vi "Main.vi"(10 "DMM Port":refnum<visa-resource-name>, 11 "Module Admin":refnum<class "Delacor_lib_QMH_Module Admin.lvclass">) -> ()   [LabVIEW 2018, in "DMM Module.lvlib"]
doc: "This template is based off of the Queued Message Handler design pattern and the Queued Message Handler project template that ships with LabVIEW.\n\nThe main difference is that the queue is private to this module and communication between modules is performed via Broadcast and Request events.\n\nRequest events are wrapped in public API methods and are handled in the Event Handling Loop (EHL) of this VI. Any module can register for Broadcast events sent by this module. The EHL generates messages based on user interface actions.\n\nThe Message Handling Loop (MHL) processes messages generated by the EHL, or by other messages. The messages are string values, so new messages can be added easily to the Message Cases case structure in the MHL. Each message cluster can also provide an optional value for Message Data, which is a variant that can be converted to whatever message-specific data is required.\n_____\nBased on DQMH Project Template 6.0.0.91."
uses:
  DMM Module.lvlib
  <vilib>/Delacor/Delacor QMH/Libraries/Module Admin_class/Delacor_lib_QMH_Module Admin.lvclass
  Module Data--cluster.ctl
  config channel Argument--cluster.ctl
  <vilib>/Delacor/Delacor QMH/Libraries/Message Queue_class/Delacor_lib_QMH_Message Queue.lvclass/Delacor_lib_QMH_Message Queue.ctl
  DMM init Argument--cluster.ctl
  Read DCV_DCI Argument--cluster.ctl
  Read DCV_DCI (Reply Payload)--cluster.ctl
  DMM Close Argument--cluster.ctl
  DMM connect and reset Argument--cluster.ctl
  DMM reset Argument--cluster.ctl
  Stop Argument--cluster.ctl
  <vilib>/Delacor/Delacor QMH/Libraries/Module Admin_class/Delacor_lib_QMH_Module Admin.lvclass/Delacor_lib_QMH_Module Admin.ctl
  Query func Argument--cluster.ctl
  Query func (Reply Payload)--cluster.ctl
  query range Argument--cluster.ctl
  query range (Reply Payload)--cluster.ctl
  <vilib>/Utility/miscctls.llb/LVPointTypeDef.ctl
  <vilib>/Delacor/Delacor QMH/Libraries/Message Queue_class/Delacor_lib_QMH_Enqueue Message (Single).vi
  <vilib>/Delacor/Delacor QMH/Libraries/Module Admin_class/Delacor_lib_QMH_Get External Launch.vi
  <vilib>/Utility/error.llb/Error Cluster From Error Code.vi
  <vilib>/ErrorRing/Error Ring.xnode
  <vilib>/Delacor/Delacor QMH/Libraries/Message Queue_class/Delacor_lib_QMH_Message Queue.lvclass
  <instrlib>/DMM4/DMM4.lvlib
panel:
  in  "DMM reset":bool
  in  "Sets to Display":u16(ring)=2 items=["1st Display", "2nd Display", "1st & 2nd Display"]
  out "DCI":dbl
  out "DCV":dbl
  in  "Read DCV, DCI Dual mode":bool
  in  "Config Channel":bool
  in  "Detector Rate":u8(ring)=1 items=["SLOW", "MID", "FAST"]
  in  "DCI Range":dbl=1.0
  in  "DCV Range":dbl=1000.0
  in  "Open&Init":bool caption="Open&init"
  out "error out":errorcluster
  out "Status":string
  in  "Simulate MHL Error":bool
  in  "Simulate EHL Error":bool
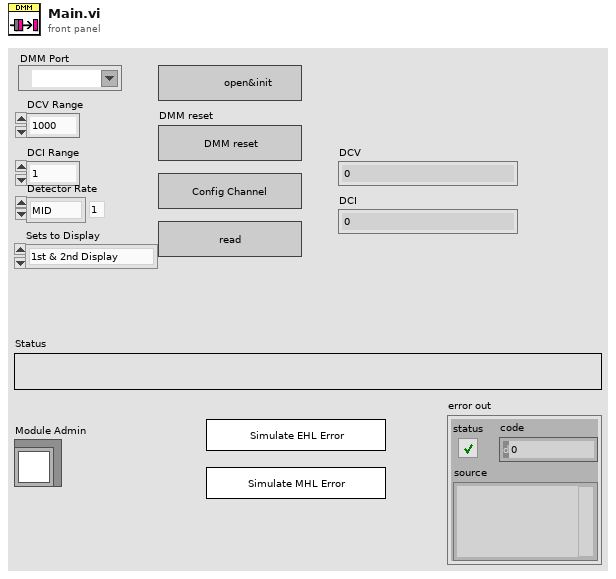
[diagram p1: front panel]
types:
  T1 = typedef "DMM Module.lvlib/Request Events--cluster.ctl" = cluster{"Stop Module":refnum<user-event>, "Do Something Else":refnum<user-event>, "Do Something Else and Wait for Reply":refnum<user-event>, "Show Panel":refnum<user-event>, "Hide Panel":refnum<user-event>, "Get Module Execution Status":refnum<user-event>, "Show Diagram":refnum<user-event>, "DMM init":refnum<user-event>, "config channel":refnum<user-event>, "Read DCV_DCI":refnum<user-event>, "DMM Close":refnum<user-event>, "DMM connect and reset":refnum<user-event>, "DMM reset":refnum<user-event>, "Query func":refnum<user-event>, "query range":refnum<user-event>}
  T2 = typedef "DMM Module.lvlib/Module Data--cluster.ctl" = cluster{"Status":string, "DMM  name":refnum<visa-resource-name>}
  T3 = typedef "DMM Module.lvlib/config channel Argument--cluster.ctl" = cluster{"Boolean":bool, "DCV range":dbl, "DCI range ":dbl, "Detector Rate":u8}
  T4 = typedef "DMM Module.lvlib/DMM init Argument--cluster.ctl" = cluster{"VISA resource name":refnum<visa-resource-name>}
  T5 = typedef "DMM Module.lvlib/Read DCV_DCI Argument--cluster.ctl" = cluster{"Wait Notifier":refnum<notifier>, "wait for reply":bool, "Sets to Display":u16}
  T6 = typedef "DMM Module.lvlib/DMM Close Argument--cluster.ctl" = cluster{"Boolean":bool}
  T7 = typedef "DMM Module.lvlib/DMM connect and reset Argument--cluster.ctl" = cluster{"Boolean":bool}
  T8 = typedef "DMM Module.lvlib/DMM reset Argument--cluster.ctl" = cluster{"Boolean":bool}
  T9 = enum32{"invalid lock state", "Not Locked", "Locked (No Password)", "Password-protected"}
  T10 = typedef "DMM Module.lvlib/Stop Argument--cluster.ctl" = cluster{"Origin":string, "Exit via Stop Module Req?":bool, "Wait for Module to stop?":bool}
  T11 = typedef "DMM Module.lvlib/Query func Argument--cluster.ctl" = cluster{"Wait Notifier":refnum<notifier>, "wait for reply":bool}
  T12 = typedef "DMM Module.lvlib/query range Argument--cluster.ctl" = cluster{"Wait Notifier":refnum<notifier>, "wait for reply":bool}
  T13 = typedef "LVPointTypeDef.ctl" = cluster{"Horizontal":i16, "Vertical":i16}
  T14 = enum32{"Invalid", "Standard", "Closed", "Hidden", "Minimized", "Maximized"}
  T15 = typedef "DMM Module.lvlib/Read DCV_DCI (Reply Payload)--cluster.ctl" = cluster{"DCV(Volts)":dbl, "DCI(mA)":dbl, "Read DCV_DCI_error":errorcluster}
  T16 = typedef "DMM Module.lvlib/Query func (Reply Payload)--cluster.ctl" = cluster{"String":string, "Query func_error":errorcluster}
  T17 = typedef "DMM Module.lvlib/query range (Reply Payload)--cluster.ctl" = cluster{"String":string, "query range_error":errorcluster}
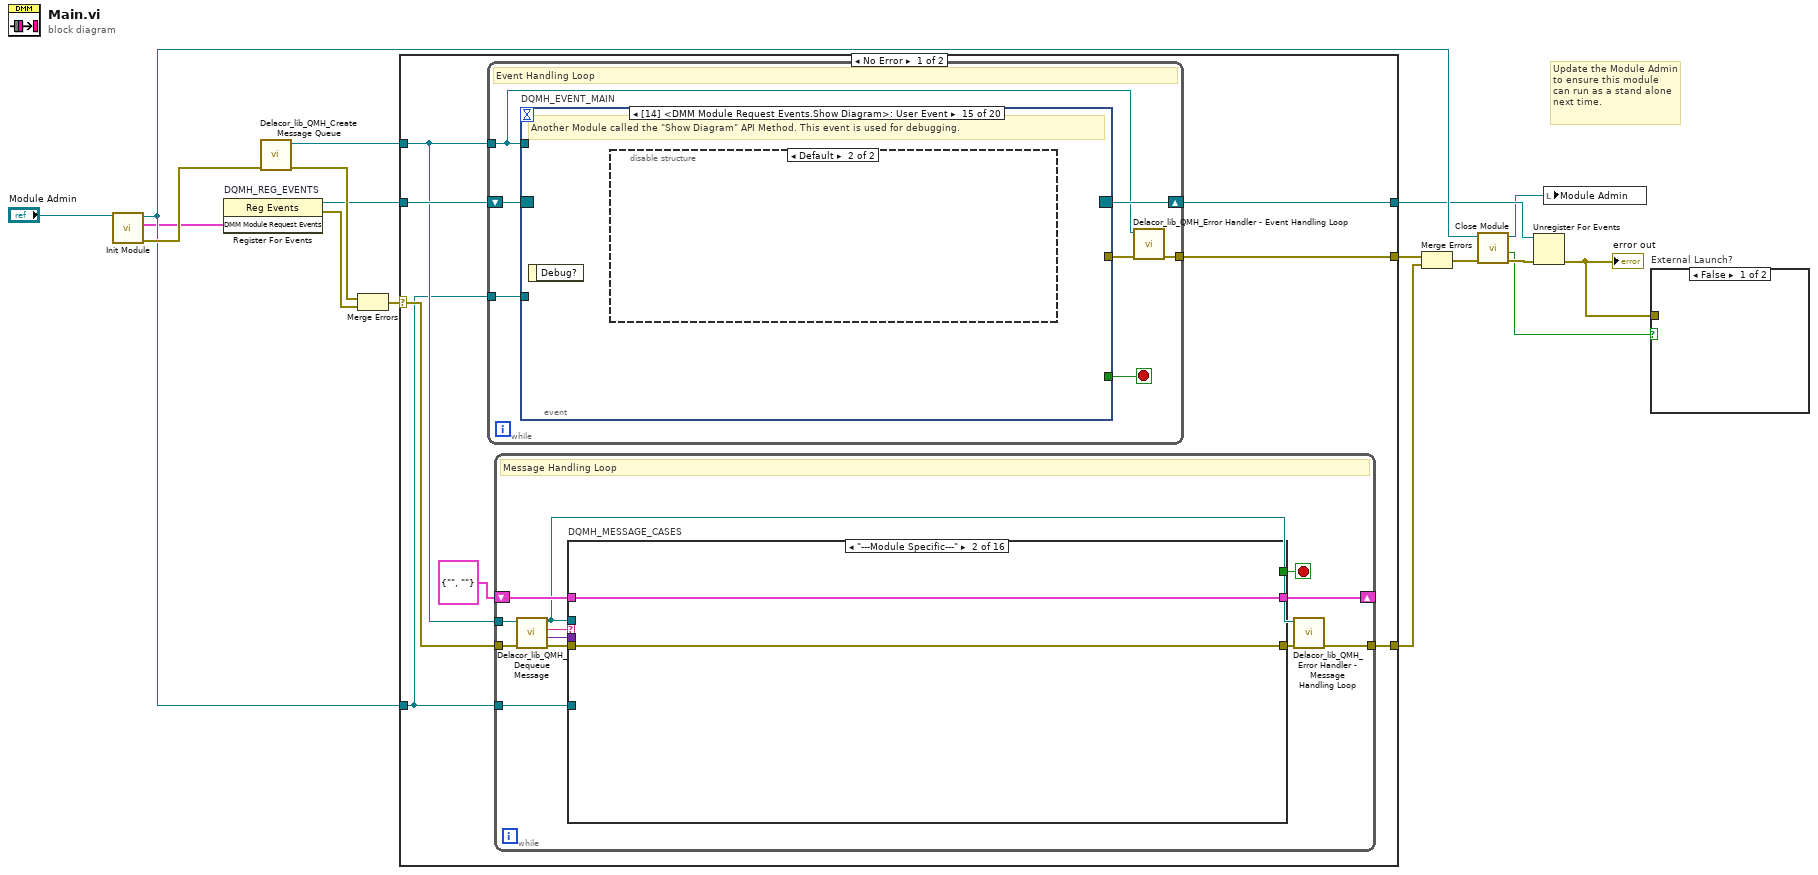
[diagram p0: block diagram]
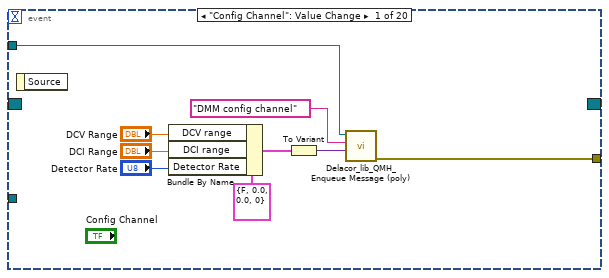
[diagram p2: hidden frame]
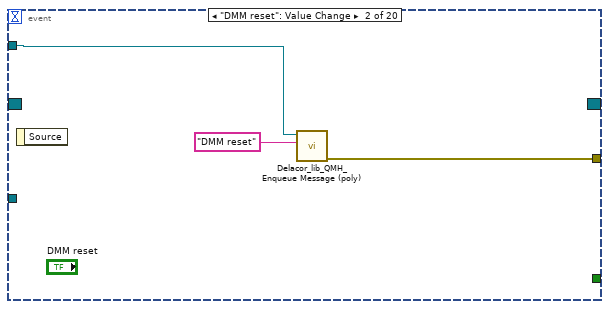
[diagram p3: hidden frame]
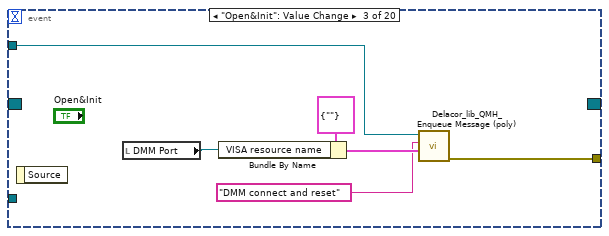
[diagram p4: hidden frame]
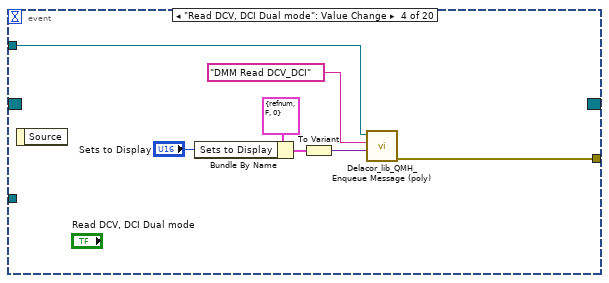
[diagram p5: hidden frame]
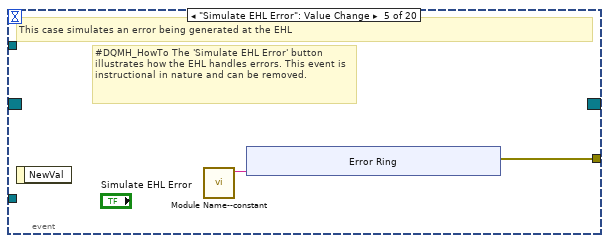
[diagram p6: hidden frame]
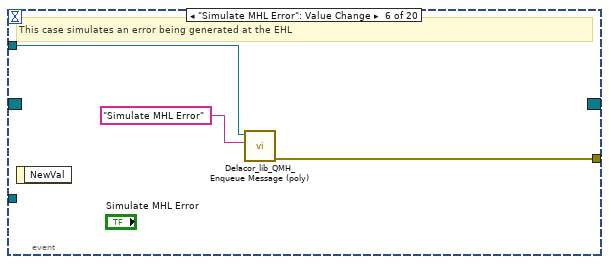
[diagram p7: hidden frame]
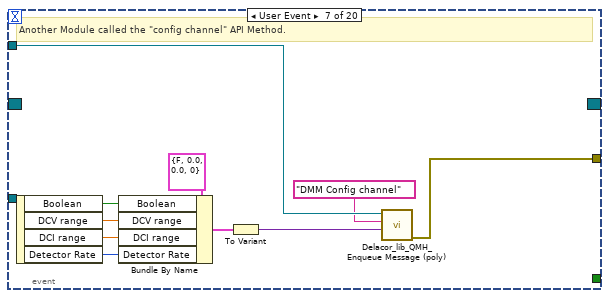
[diagram p8: hidden frame]
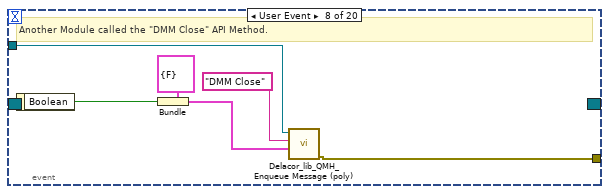
[diagram p9: hidden frame]
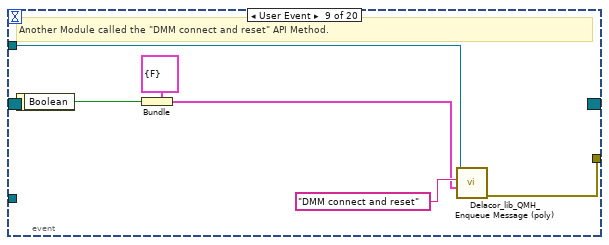
[diagram p10: hidden frame]
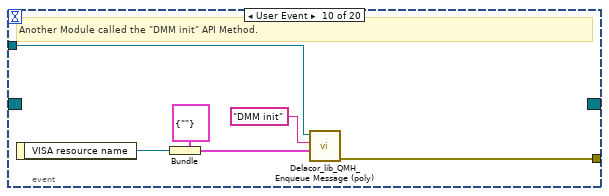
[diagram p11: hidden frame]
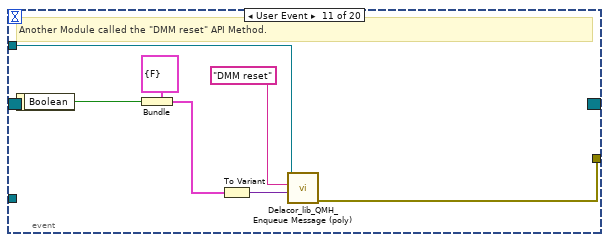
[diagram p12: hidden frame]
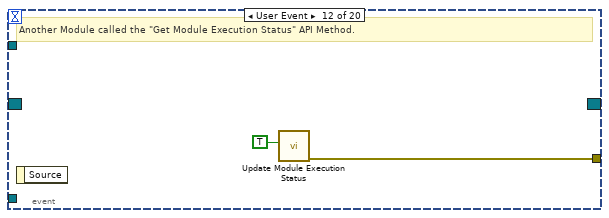
[diagram p13: hidden frame]
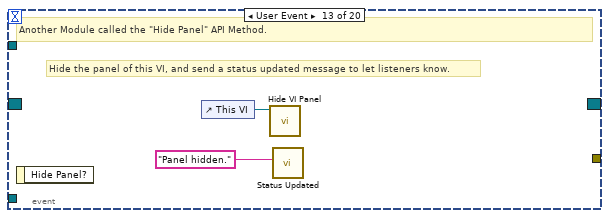
[diagram p14: hidden frame]
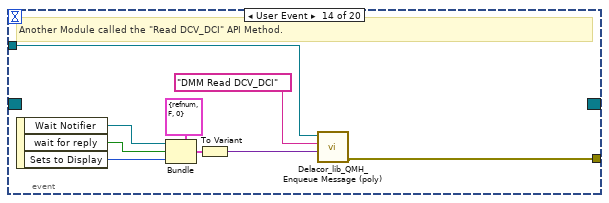
[diagram p15: hidden frame]
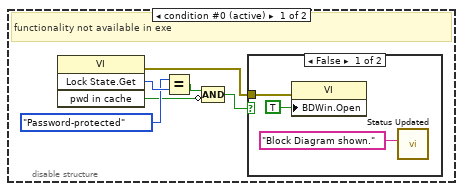
[diagram p16: hidden frame]
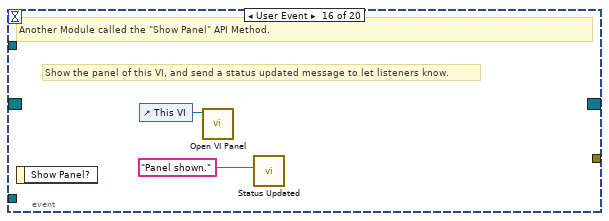
[diagram p18: hidden frame]
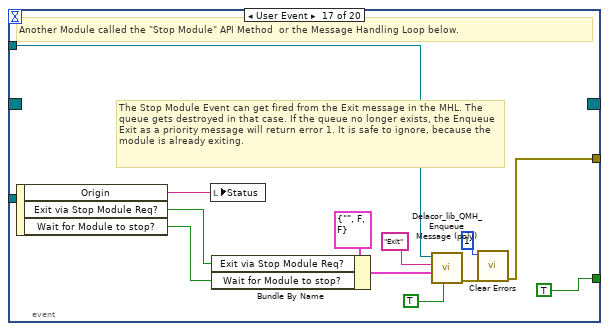
[diagram p19: hidden frame]
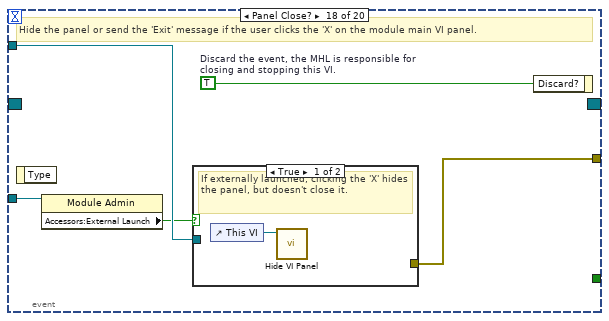
[diagram p20: hidden frame]
diagram:
  # "Update the Module Admin to ensure this module can run as a stand alone next time."
  n1 = call "Init Module.vi"("Singleton Module Admin in"="Module Admin") -> ("error out"=w16:errorcluster, "DMM Module Request Events"=w5:T1, "Singleton Module Admin out"=w8:refnum<class "Delacor_lib_QMH_Module Admin.lvclass">)  [unwired: 8 in]
  n2 = register-events "DQMH_REG_EVENTS"(w5) -> (reference out=w6:refnum<event-registration>, error out=w9:errorcluster)  [unwired: 2 in]
  n3 = call <vilib>:"Delacor_lib_QMH_Create Message Queue.vi"("error in"=w16) -> ("error out"=w11:errorcluster, "Message Queue"=w4:refnum<class "Delacor_lib_QMH_Message Queue.lvclass">)  [unwired: 9 in]
  n4 = Merge Errors(w11, w9) -> (w10:errorcluster)
  n5 = case shown="No Error" w10 {
    selector: w10 -> [w23 w418]
    tunnel: [w25 w417] -> w17
    tunnel: [w22 w423] -> w7
    tunnel: w6 -> [w20 w423]
    tunnel: w4 -> [w19 w416]
    tunnel: [w24 _] -> w14
    tunnel: w8 -> [w18 w419]
    frame No Error {
      n6 = while {
        tunnel: w19 -> [w26]
        shift-right: [w29] -> w22
        shift-left: w20 -> [w30]
        tunnel: [w31] -> w24
        tunnel: w18 -> [w27]
        stop <- w28 stop-if-true
        # "Event Handling Loop"
        n7 = event "DQMH_EVENT_MAIN" shown="[14] <DMM Module Request Events.Show Diagram>: User Event" {
          selector: w30 -> [_ _ _ _ _ _ _ _ _ _ _ _ _ _ _ _ _ _ _ _]
          dyn-events: [_ _ _ _ _ _ _ _ _ _ _ _ _ _ _ _ _ _ _ _] -> w29
          timeout: _ -> [_ _ _ _ _ _ _ _ _ _ _ _ _ _ _ _ _ _ _ _]
          tunnel: [_ _ _ _ _ _ _ _ _ _ _ _ _ _ _ _ TRUE ("Discard?") _ _ _] -> w28
          tunnel: w26 -> [w36 w44 w50 w57 _ w68 w79 w85 w91 w97 w104 _ _ w117 _ _ w129 w143 w157 w164]
          tunnel: [w35 w42 w47 w52 w59 w69 w75 w80 w86 w92 w100 w106 _ w111 _ _ w139 w145 w151 w158] -> w32
          tunnel: w27 -> [_ _ _ _ _ _ _ _ _ _ _ _ _ _ _ _ _ w142 _ _]
          event "Config Channel": Value Change {
            n8 = event-data() -> ()  [unwired: 1 in, 1 out]
            n9 = Bundle By Name(cluster=T3 {"Boolean"=FALSE, "DCV range"=0.0, "DCI range "=0.0, "Detector Rate"=0} ("config channel Argument"), "DCV range"="DCV Range", "DCI range"="DCI Range", "Detector Rate"="Detector Rate") -> (w34:T3)
            n10 = To Variant(anything=w34) -> (Variant=w33:variant)
            n11 = call-poly <vilib>:"Delacor_lib_QMH_Enqueue Message (poly).vi"("Message Data"=w33, "Message"="DMM config channel", "Message Queue in"=w36) -> ("error out"=w35:errorcluster)  [unwired: 7 in, 1 out]
          }
          event "DMM reset": Value Change {
            n12 = event-data() -> ()  [unwired: 1 in, 1 out]
            n13 = call-poly <vilib>:"Delacor_lib_QMH_Enqueue Message (poly).vi"("Message"="DMM reset", "Message Queue in"=w44) -> ("error out"=w42:errorcluster)  [unwired: 8 in, 1 out]
          }
          event "Open&Init": Value Change {
            n14 = event-data() -> ()  [unwired: 1 in, 1 out]
            n15 = local read "DMM Port"() -> (w46:refnum<visa-resource-name>)
            n16 = Bundle By Name(cluster=T4 {"VISA resource name"=""} ("DMM init Argument"), "VISA resource name"=w46) -> (w48:T4)
            n17 = call-poly <vilib>:"Delacor_lib_QMH_Enqueue Message (poly).vi"("Message Data"=w48, "Message"="DMM connect and reset", "Message Queue in"=w50) -> ("error out"=w47:errorcluster)  [unwired: 7 in, 1 out]
          }
          event "Read DCV, DCI Dual mode": Value Change {
            n18 = event-data() -> ()  [unwired: 1 in, 1 out]
            n19 = Bundle By Name(cluster=T5 {"Wait Notifier"=refnum, "wait for reply"=FALSE, "Sets to Display"=0} ("Read DCV_DCI Argument"), "Sets to Display"="Sets to Display") -> (w53:T5)
            n20 = To Variant(anything=w53) -> (Variant=w51:variant)
            n21 = call-poly <vilib>:"Delacor_lib_QMH_Enqueue Message (poly).vi"("Message Data"=w51, "Message"="DMM Read DCV_DCI", "Message Queue in"=w57) -> ("error out"=w52:errorcluster)  [unwired: 7 in, 1 out]
          }
          event "Simulate EHL Error": Value Change {
            # "#DQMH_HowTo The 'Simulate EHL Error' button  illustrates how the EHL handles errors. This event is instructional in nature and can be removed."
            # "This case simulates an error being generated at the EHL"
            n22 = event-data() -> ()  [unwired: 1 in, 1 out]
            n23 = call "Module Name--constant.vi"() -> ("Module Name"=w58:string)  [unwired: 11 in]
            n24 = xnode "Error Ring"("parameter 0"=w58) -> ("error out"=w59:errorcluster)
          }
          event "Simulate MHL Error": Value Change {
            # "This case simulates an error being generated at the EHL"
            n25 = event-data() -> ()  [unwired: 1 in, 1 out]
            n26 = call-poly <vilib>:"Delacor_lib_QMH_Enqueue Message (poly).vi"("Message"="Simulate MHL Error", "Message Queue in"=w68) -> ("error out"=w69:errorcluster)  [unwired: 8 in, 1 out]
          }
          event User Event {
            # "Another Module called the \"config channel\" API Method."
            n27 = event-data() -> ("Boolean"=w76:bool, "DCV range"=w74:dbl, "DCI range"=w73:dbl, "Detector Rate"=w72:u8)  [unwired: 1 in]
            n28 = Bundle By Name(cluster=T3 {"Boolean"=FALSE, "DCV range"=0.0, "DCI range "=0.0, "Detector Rate"=0} ("config channel Argument"), "Boolean"=w76, "DCV range"=w74, "DCI range"=w73, "Detector Rate"=w72) -> (w71:T3)
            n29 = To Variant(anything=w71) -> (Variant=w70:variant)
            n30 = call-poly <vilib>:"Delacor_lib_QMH_Enqueue Message (poly).vi"("Message Data"=w70, "Message"="DMM Config channel", "Message Queue in"=w79) -> ("error out"=w75:errorcluster)  [unwired: 7 in, 1 out]
          }
          event User Event {
            # "Another Module called the \"DMM Close\" API Method."
            n31 = event-data() -> ("Boolean"=w81:bool)  [unwired: 1 in]
            n32 = Bundle(cluster=T6 {"Boolean"=FALSE} ("DMM Close Argument"), "Boolean"=w81) -> (w82:T6)
            n33 = call-poly <vilib>:"Delacor_lib_QMH_Enqueue Message (poly).vi"("Message Data"=w82, "Message"="DMM Close", "Message Queue in"=w85) -> ("error out"=w80:errorcluster)  [unwired: 7 in, 1 out]
          }
          event User Event {
            # "Another Module called the \"DMM connect and reset\" API Method."
            n34 = event-data() -> ("Boolean"=w87:bool)  [unwired: 1 in]
            n35 = Bundle(cluster=T7 {"Boolean"=FALSE} ("DMM connect and reset Argument"), "Boolean"=w87) -> (w88:T7)
            n36 = call-poly <vilib>:"Delacor_lib_QMH_Enqueue Message (poly).vi"("Message Data"=w88, "Message"="DMM connect and reset", "Message Queue in"=w91) -> ("error out"=w86:errorcluster)  [unwired: 7 in, 1 out]
          }
          event User Event {
            # "Another Module called the \"DMM init\" API Method."
            n37 = event-data() -> ("VISA resource name"=w93:refnum<visa-resource-name>)  [unwired: 1 in]
            n38 = Bundle(cluster=T4 {"VISA resource name"=""} ("DMM init Argument"), "VISA resource name"=w93) -> (w94:T4)
            n39 = call-poly <vilib>:"Delacor_lib_QMH_Enqueue Message (poly).vi"("Message Data"=w94, "Message"="DMM init", "Message Queue in"=w97) -> ("error out"=w92:errorcluster)  [unwired: 7 in, 1 out]
          }
          event User Event {
            # "Another Module called the \"DMM reset\" API Method."
            n40 = event-data() -> ("Boolean"=w101:bool)  [unwired: 1 in]
            n41 = Bundle(cluster=T8 {"Boolean"=FALSE} ("DMM reset Argument"), "Boolean"=w101) -> (w99:T8)
            n42 = To Variant(anything=w99) -> (Variant=w98:variant)
            n43 = call-poly <vilib>:"Delacor_lib_QMH_Enqueue Message (poly).vi"("Message Data"=w98, "Message"="DMM reset", "Message Queue in"=w104) -> ("error out"=w100:errorcluster)  [unwired: 7 in, 1 out]
          }
          event User Event {
            # "Another Module called the \"Get Module Execution Status\" API Method."
            n44 = event-data() -> ()  [unwired: 1 in, 1 out]
            n45 = call "Update Module Execution Status.vi"("Running?"=TRUE) -> ("error out"=w106:errorcluster)  [unwired: 10 in]
          }
          event User Event {
            # "Hide the panel of this VI, and send a status updated message to let listeners know."
            # "Another Module called the \"Hide Panel\" API Method."
            n46 = event-data() -> ()  [unwired: 1 in, 1 out]
            n47 = control-ref of="This VI"() -> (w108:refnum<vi>)
            n48 = call "Hide VI Panel.vi"("VI"=w108) -> ()  [unwired: 10 in, 1 out]
            n49 = call "Status Updated.vi"("Status"="Panel hidden." ("format string")) -> ()  [unwired: 10 in, 1 out]
          }
          event User Event {
            # "Another Module called the \"Read DCV_DCI\" API Method."
            n50 = event-data() -> ("Wait Notifier"=w113:refnum<notifier>, "wait for reply"=w112:bool, "Sets to Display"=w110:u16)  [unwired: 1 in]
            n51 = Bundle(cluster=T5 {"Wait Notifier"=refnum, "wait for reply"=FALSE, "Sets to Display"=0} ("Read DCV_DCI Argument"), "Wait Notifier"=w113, "wait for reply"=w112, "Sets to Display"=w110) -> (w114:T5)
            n52 = To Variant(anything=w114) -> (Variant=w109:variant)
            n53 = call-poly <vilib>:"Delacor_lib_QMH_Enqueue Message (poly).vi"("Message Data"=w109, "Message"="DMM Read DCV_DCI", "Message Queue in"=w117) -> ("error out"=w111:errorcluster)  [unwired: 7 in, 1 out]
          }
          event User Event {
            # "Another Module called the \"Show Diagram\" API Method. This event is used for debugging."
            n54 = event-data() -> ()  [unwired: 1 in, 1 out]
            n55 = disable-structure shown="Default" {
              frame condition #0 (active) {
                # "functionality not available in exe"
                n56 = invoke class="VI" method="Lock State.Get"() -> (error out=w123:errorcluster, "Get Lock State"=w122:T9, "pwd in cache"=w119:bool)  [unwired: 4 in, 1 out]
                n57 = Equal?(x=T9."Password-protected", y=w122) -> (x = y?=w120:bool)
                n58 = Compound Arithmetic op=AND(w120, invert w119) -> (w118:bool)
                n59 = case shown="False" w118 {
                  tunnel: w123 -> [w126 _]
                  frame False {
                    n60 = property class="VI"(error in=w126, "BDWin.Open"=TRUE ("Block Diagram Window:Open")) -> ()  [unwired: 1 in, 2 out]
                    n61 = call "Status Updated.vi"("Status"="Block Diagram shown." ("format string")) -> ()  [unwired: 10 in, 1 out]
                  }
                  frame True {
                    # "Password-protected VI, and the password is not in the cache. Do not show the diagram."
                  }
                }
              }
              frame condition #1 {
              }
            }
          }
          event User Event {
            # "Show the panel of this VI, and send a status updated message to let listeners know."
            # "Another Module called the \"Show Panel\" API Method."
            n62 = event-data() -> ()  [unwired: 1 in, 1 out]
            n63 = control-ref of="This VI"() -> (w128:refnum<vi>)
            n64 = call "Open VI Panel.vi"("VI"=w128) -> ()  [unwired: 10 in, 1 out]
            n65 = call "Status Updated.vi"("Status"="Panel shown." ("format string")) -> ()  [unwired: 10 in, 1 out]
          }
          event User Event {
            # "The Stop Module Event can get fired from the Exit message in the MHL. The queue gets destroyed in that case. If the queue no longer exists, the Enqueue Exit as a priority message will return error 1. It is safe to ignore, because the module is already exiting."
            # "Another Module called the \"Stop Module\" API Method  or the Message Handling Loop below."
            n66 = event-data() -> ("Origin"=w136:string, "Exit via Stop Module Req?"=w132:bool, "Wait for Module to stop?"=w131:bool)  [unwired: 1 in]
            n67 = local write "Status"(w136) -> ()
            n68 = Bundle By Name(cluster=T10 {"Origin"="", "Exit via Stop Module Req?"=FALSE, "Wait for Module to stop?"=FALSE} ("Stop Argument"), "Exit via Stop Module Req?"=w132, "Wait for Module to stop?"=w131) -> (w130:T10)
            n69 = call-poly <vilib>:"Delacor_lib_QMH_Enqueue Message (poly).vi"("Priority Message? (F)"=TRUE, "Message Data"=w130, "Message"="Exit", "Message Queue in"=w129) -> ("error out"=w140:errorcluster)  [unwired: 6 in, 1 out]
            n70 = call <vilib>:"Clear Errors.vi"("error in (no error)"=w140, "specific error code to clear (0: all)"=1) -> ("error out"=w139:errorcluster)  [unwired: 4 in, 1 out]
          }
          event Panel Close? {
            w144 = TRUE  # Discard the event, the MHL is responsible for closing and stopping this VI.
            # "Hide the panel or send the 'Exit' message if the user clicks the 'X' on the module main VI panel."
            n71 = event-data() -> ()  [unwired: 1 in, 1 out]
            n72 = property class="Module Admin"(reference=w142) -> ("Accessors:External Launch"=w141:bool)  [unwired: 1 in, 2 out]
            n73 = case shown="True" w141 {
              tunnel: w143 -> [_ w149]
              tunnel: [_ w150] -> w145
              frame True {
                # "If externally launched, clicking the 'X' hides the panel, but doesn't close it."
                n74 = control-ref of="This VI"() -> (w146:refnum<vi>)
                n75 = call "Hide VI Panel.vi"("VI"=w146) -> ()  [unwired: 10 in, 1 out]
              }
              frame False {
                # "If run as a stand-alone VI, clicking the panel 'X' stops the VI."
                n76 = call-poly <vilib>:"Delacor_lib_QMH_Enqueue Message (poly).vi"("Priority Message? (F)"=TRUE, "Message"="Exit", "Message Queue in"=w149) -> ("error out"=w150:errorcluster)  [unwired: 7 in, 1 out]
              }
            }
            n77 = event-data("Discard?"=w144) -> ()  [unwired: 1 in, 1 out]
          }
          event User Event {
            # "Another Module called the \"Query func\" API Method."
            n78 = event-data() -> ("Wait Notifier"=w153:refnum<notifier>, "wait for reply"=w152:bool)  [unwired: 1 in]
            n79 = Bundle(cluster=T11 {"Wait Notifier"=refnum, "wait for reply"=FALSE} ("Query func Argument"), "Wait Notifier"=w153, "wait for reply"=w152) -> (w154:T11)
            n80 = call-poly <vilib>:"Delacor_lib_QMH_Enqueue Message (poly).vi"("Message Data"=w154, "Message"="Query func", "Message Queue in"=w157) -> ("error out"=w151:errorcluster)  [unwired: 7 in, 1 out]
          }
          event User Event {
            # "Another Module called the \"query range\" API Method."
            n81 = event-data() -> ("Wait Notifier"=w160:refnum<notifier>, "wait for reply"=w159:bool)  [unwired: 1 in]
            n82 = Bundle(cluster=T12 {"Wait Notifier"=refnum, "wait for reply"=FALSE} ("query range Argument"), "Wait Notifier"=w160, "wait for reply"=w159) -> (w161:T12)
            n83 = call-poly <vilib>:"Delacor_lib_QMH_Enqueue Message (poly).vi"("Message Data"=w161, "Message"="query range", "Message Queue in"=w164) -> ("error out"=w158:errorcluster)  [unwired: 7 in, 1 out]
          }
        }
        n84 = call-dynamic "Delacor_lib_QMH_Error Handler - Event Handling Loop.vi"("error in"=w32, "Message Queue in"=w26) -> ("dup error in"=w31:errorcluster)  [unwired: 8 in, 1 out]
      }
      n85 = while {
        tunnel: w19 -> [w167]
        shift-right: [w171] -> _
        shift-left: T2 {"Status"="", "DMM  name"=""} ("Data Cluster") -> [w172]
        tunnel: w23 -> [w175]
        tunnel: [w173] -> w25
        tunnel: w18 -> [w165]
        stop <- w170 stop-if-true
        # "Message Handling Loop"
        n86 = call-dynamic "Delacor_lib_QMH_Dequeue Message.vi"("error in"=w175, "Message Queue in"=w167) -> ("error out"=w174:errorcluster, "Message Data"=w168:variant, "Message"=w169:string, "Message Queue out"=w166:refnum<class "Delacor_lib_QMH_Message Queue.lvclass">)  [unwired: 6 in]
        n87 = case "DQMH_MESSAGE_CASES" shown="\"---Module Specific---\"" w169 {
          selector: w169 -> [_ _ _ _ _ _ _ _ _ _ _ _ _ _ _ w403]
          tunnel: w166 -> [_ _ _ _ _ _ _ _ _ _ _ _ _ w368 w390 _]
          tunnel: w174 -> [w195 w199 w206 w222 w232 w241 w257 w288 w325 w346 w349 w352 w357 w374 w396 w405]
          tunnel: [w179 w199 w201 w217 w229 w234 w253 w279 w316 w337 w349 w352 w356 w371 w393 w406] -> w176
          tunnel: w172 -> [w181 w198 w203 w219 w228 w237 w247 w278 w315 w336 w350 w351 w354 w370 w382 w404]
          tunnel: [w177 w198 w203 w219 w228 w237 w247 w278 w315 w336 w350 w351 w354 w370 w382 w404] -> w171
          tunnel: [_ _ _ _ _ _ _ _ _ _ _ _ _ _ w389 _] -> w170
          tunnel: w168 -> [_ _ w205 w221 w231 w240 w256 w286 w323 w344 _ _ _ w369 w388 _]
          tunnel: w165 -> [w188 _ _ _ _ _ _ _ _ _ _ _ _ w367 w383 _]
          frame "Initialize" {
            w178 = "Initial Message" ("Initial Message")
            # "Initialize - Any operation that needs to be done before the module can receive messages. Synchronize Caller Events.vi will inform Start Module.vi that the module has launched and is ready to receive messages. Module Did Init.vi will broadcast that the module initialized."
            n88 = call "Synchronize Caller Events.vi"("error in (no error)"=w195, "Singleton Module Admin in"=w188) -> ("error out"=w183:errorcluster, "Singleton Module Admin out"=w185:refnum<class "Delacor_lib_QMH_Module Admin.lvclass">)  [unwired: 8 in]
            n89 = property class="Module Admin"(reference=w185) -> ("Accessors:External Launch"=w182:bool)  [unwired: 1 in, 2 out]
            n90 = call "Module Name--constant.vi"() -> ("Module Name"=w194:string)  [unwired: 11 in]
            n91 = Select(t=T14."Hidden" ("State"), s=w182, f=T14."Standard" ("State")) -> (s? t:f=w189:T14)
            n92 = property class="VI"("Front Panel.Title"=w194) -> (reference out=w193:refnum<vi>, error out=w197:errorcluster)  [unwired: 2 in]
            n93 = invoke class="VI" method="FP.Open"(reference=w193, error in=w197, "State"=w189) -> (reference out=w192:refnum<vi>, error out=w196:errorcluster)  [unwired: 2 in, 3 out]
            n94 = Bundle By Name(cluster=w181, "DMM  name"="DMM Port", "Status"=w178) -> (w177:T2)
            n95 = invoke class="VI" method="FP.Center"(reference=w192, error in=w196) -> ()  [unwired: 1 in, 3 out]
            n96 = property on="Pane" class="Pane"("Origin"=T13 {"Horizontal"=0, "Vertical"=0}) -> ()  [unwired: 2 in, 2 out]
            n97 = call "Module Name--constant.vi"() -> ("Module Name"=w186:string)  [unwired: 11 in]
            n98 = call "Module Did Init.vi"("error in (no error)"=w183, "Initialized?"=TRUE, "Origin"=w186) -> ("error out"=w179:errorcluster)  [unwired: 8 in]
            "Status" <- w178
          }
          frame "---Module Specific---" {
            # "Separator -- The following cases handle messages specific to this Module."
          }
          frame "DMM connect and reset" {
            # "Connect DMM and reset DMM"
            n99 = Variant To Data(error in=w206, type=T7 {"Boolean"=FALSE} ("DMM connect and reset Argument"), Variant=w205) -> (error out=w202:errorcluster)  [unwired: 1 out]
            n100 = disable-structure shown="Default" {
              disable-tunnel: w203 -> [w210 _]
              disable-tunnel: [w208 _] -> w200
              frame condition #0 (active) {
                w211 = u32 115200 items=["9600"=9600, "19200"=19200, "38400"=38400, "57600"=57600, "115200"=115200] ("Configure RS232 Baud Rate")
                n101 = Unbundle By Name(w210) -> ("DMM  name"=w209:refnum<visa-resource-name>)
                n102 = call <instrlib>:"Initialize.vi"("Configure RS232 Baud Rate"=w211, "VISA resource name"=w209) -> ("error out"=w213:errorcluster, "VISA resource name out"=w212:refnum<visa-resource-name>)  [unwired: 6 in, 2 out]
                n103 = call <instrlib>:"Reset.vi"("error in (no error)"=w213, "VISA resource name"=w212) -> ("error out"=w207:errorcluster)  [unwired: 8 in, 1 out]
                n104 = flat-sequence {
                  tunnel: [w214] -> w208
                  tunnel: w207 -> [w214]
                  frame #0 {
                    n105 = Wait (ms)(milliseconds to wait=u32 200) -> ()  [unwired: 1 out]
                  }
                }
              }
              frame condition #1 {
              }
            }
            n106 = Merge Errors(w202, w200) -> (w201:errorcluster)
          }
          frame "DMM Close" {
            # "Close COMport to DMM"
            n107 = disable-structure shown="Default" {
              disable-tunnel: w219 -> [w227 _]
              disable-tunnel: [w226 _] -> w216
              frame condition #0 (active) {
                n108 = Unbundle By Name(w227) -> ("DMM  name"=w225:refnum<visa-resource-name>)
                n109 = call <instrlib>:"Reset.vi"("VISA resource name"=w225) -> ("error out"=w223:errorcluster, "VISA resource name out"=w224:refnum<visa-resource-name>)  [unwired: 9 in]
                n110 = call <instrlib>:"Close.vi"("error in (no error)"=w223, "VISA resource name"=w224) -> ("error out"=w226:errorcluster)  [unwired: 9 in]
              }
              frame condition #1 {
              }
            }
            n111 = Variant To Data(error in=w222, type=T6 {"Boolean"=FALSE} ("DMM Close Argument"), Variant=w221) -> (error out=w218:errorcluster)  [unwired: 1 out]
            n112 = Merge Errors(w218, w216) -> (w217:errorcluster)
          }
          frame "DMM init" {
            # "#Hung_comment :\nNo longer use"
            # "Open port and initialize DMM  and reset DMM"
            n113 = Variant To Data(error in=w232, type=T4 {"VISA resource name"=""} ("DMM init Argument"), Variant=w231) -> (error out=w229:errorcluster)  [unwired: 1 out]
          }
          frame "DMM reset" {
            # "Reset Measurement Mode"
            n114 = Variant To Data(error in=w241, type=T8 {"Boolean"=FALSE} ("DMM reset Argument"), Variant=w240) -> (data=w238:T8, error out=w236:errorcluster)
            n115 = Unbundle By Name(w238) -> ()  [unwired: 1 out]
            n116 = disable-structure shown="Default" {
              disable-tunnel: w237 -> [w244 _]
              disable-tunnel: [w242 _] -> w235
              frame condition #0 (active) {
                n117 = Unbundle By Name(w244) -> ("DMM  name"=w243:refnum<visa-resource-name>)
                n118 = call <instrlib>:"Reset.vi"("VISA resource name"=w243) -> ("error out"=w242:errorcluster)  [unwired: 9 in, 1 out]
              }
              frame condition #1 {
              }
            }
            n119 = Merge Errors(w236, w235) -> (w233:errorcluster)
            n120 = flat-sequence {
              tunnel: [w246] -> w234
              tunnel: w233 -> [w246]
              frame #0 {
                n121 = Wait (ms)(milliseconds to wait=u32 200) -> ()  [unwired: 1 out]
              }
            }
          }
          frame "DMM Config channel" {
            # "Config DMM mode: dual measurements, CH1: DCV; CH2: DCI"
            n122 = Variant To Data(error in=w257, type=T3 {"Boolean"=FALSE, "DCV range"=0.0, "DCI range "=0.0, "Detector Rate"=0} ("config channel Argument"), Variant=w256) -> (data=w254:T3, error out=w249:errorcluster)
            n123 = Unbundle By Name(w254) -> ("Detector Rate"=w250:u8, "DCV range"=w252:dbl, "DCI range"=w251:dbl)
            n124 = disable-structure shown="Default" {
              disable-tunnel: w252 -> [w272 _]
              disable-tunnel: w251 -> [w261 _]
              disable-tunnel: w250 -> [w270 _]
              disable-tunnel: [w258 _] -> w248
              disable-tunnel: w247 -> [w264 _]
              frame condition #0 (active) {
                w262 = FALSE ("Enable Auto Range")
                w260 = u8 2 items=["DC Voltage", "AC Voltage", "DC Current", "AC Current", "2-Wire Resistance", "Frequency", "Period", "None"] ("Function")
                w266 = u8 0 items=["DC Voltage", "AC Voltage", "DC+AC Voltage", "DC Current", "AC Current", "DC+AC Current", "2-Wire Resistance", "Frequency", "Period", "Continuity", "Diode", "Temperature", "Capacitance"] ("Function")
                n125 = Unbundle By Name(w264) -> ("DMM  name"=w271:refnum<visa-resource-name>)
                n126 = call <instrlib>:"Sets and Query the Detector Rate.vi"("Enable to Query"=FALSE, "Enable to Sets"=TRUE, "Detector Rate"=w270, "VISA resource name"=w271) -> ("error out"=w265:errorcluster, "VISA resource name out"=w267:refnum<visa-resource-name>)  [unwired: 5 in, 1 out]
                n127 = call <instrlib>:"Configure the Function on 1st Display .vi"("Manual Range"=w272, "Enable Auto Range"=w262, "error in"=w265, "Function"=w266, "VISA resource name"=w267) -> ("error out"=w259:errorcluster, "VISA resource name out"=w263:refnum<visa-resource-name>)  [unwired: 5 in]
                n128 = call <instrlib>:"Configure the Function on 2nd Display.vi"("Manual Range"=w261, "Enable Auto Range"=w262, "error in"=w259, "Function"=w260, "VISA resource name"=w263) -> ("error out"=w258:errorcluster)  [unwired: 5 in, 1 out]
              }
              frame condition #1 {
              }
            }
            n129 = Merge Errors(w249, w248) -> (w253:errorcluster)
          }
          frame "DMM Read DCV_DCI" {
            # "Read DCV, DCI dual measurements"
            n130 = Variant To Data(error in=w288, type=T5 {"Wait Notifier"=refnum, "wait for reply"=FALSE, "Sets to Display"=0} ("Read DCV_DCI Argument"), Variant=w286) -> (data=w284:T5, error out=w287:errorcluster)
            n131 = Unbundle By Name(w284) -> ("Sets to Display"=w276:u16, "Wait Notifier"=w283:refnum<notifier>, "wait for reply"=w282:bool)
            n132 = Unbundle By Name(w278) -> ("DMM  name"=w277:refnum<visa-resource-name>)
            n133 = disable-structure shown="Default" {
              disable-tunnel: w277 -> [w300 _]
              disable-tunnel: w276 -> [w299 _]
              disable-tunnel: [w298 _] -> w275
              disable-tunnel: [w294 128.09] -> w274
              disable-tunnel: [w289 292.0] -> w273
              frame condition #0 (active) {
                n134 = call <instrlib>:"Returns 1st and 2nd Display Value.vi"("Sets to Display"=w299, "VISA resource name"=w300) -> ("error out"=w298:errorcluster, "Return the Value"=w296:string)  [unwired: 7 in, 1 out]
                n135 = Match Pattern(string=w296, regular expression=",") -> (before substring=w295:string, after substring=w293:string)  [unwired: 1 in, 2 out]
                n136 = Fract/Exp String To Number(string=w295) -> (number=w294:dbl)  [unwired: 3 in, 1 out]
                "DCV" <- w294
                n137 = Fract/Exp String To Number(string=w293) -> (number=w292:dbl)  [unwired: 3 in, 1 out]
                "DCI" <- w292
                n138 = Multiply(x=w292, y=1000.0) -> (x*y=w290:dbl)
                n139 = Absolute Value(x=w290) -> (abs(x)=w289:dbl)
              }
              frame condition #1 {
              }
            }
            n140 = Merge Errors(w287, w275) -> (w279:errorcluster)
            n141 = Bundle By Name(cluster=T15 {"DCV(Volts)"=0.0, "DCI(mA)"=0.0, "Read DCV_DCI_error"={"status"=FALSE, "code"=0, "source"=""}} ("Read DCV_DCI (Reply Payload)"), "DCV(Volts)"=w274, "DCI(mA)"=w273) -> (w281:T15)
            n142 = case shown="True" w282 {
              tunnel: w283 -> [_ w304]
              tunnel: w281 -> [_ w303]
              frame False {
              }
              frame True {
                n143 = Send Notification(notification=w303, notifier=w304) -> ()  [unwired: 1 in, 2 out]
              }
            }
          }
          frame "Query func" {
            w306 = u8 1 items=["1st Display", "2nd Display"] ("Query form Display")
            w313 = u8 0 items=["1st Display", "2nd Display"] ("Query form Display")
            # "Check measurement Mode  chan1"
            n144 = Variant To Data(error in=w325, type=T11 {"Wait Notifier"=refnum, "wait for reply"=FALSE} ("Query func Argument"), Variant=w323) -> (data=w321:T11, error out=w324:errorcluster)
            n145 = Unbundle By Name(w315) -> ("DMM  name"=w314:refnum<visa-resource-name>)
            n146 = Unbundle By Name(w321) -> ("Wait Notifier"=w320:refnum<notifier>, "wait for reply"=w319:bool)
            n147 = call <instrlib>:"Query the Current Function.vi"("Query form Display"=w313, "VISA resource name"=w314) -> ("error out"=w312:errorcluster, "Return the String"=w310:string, "VISA resource name out"=w311:refnum<visa-resource-name>)  [unwired: 7 in]
            n148 = call <instrlib>:"Query the Current Function.vi"("error in"=w312, "Query form Display"=w306, "VISA resource name"=w311) -> ("error out"=w305:errorcluster, "Return the String"=w308:string)  [unwired: 6 in, 1 out]
            n149 = Merge Errors(w324, w305) -> (w316:errorcluster)
            n150 = Concatenate Strings(w310, ":" ("string"), w308) -> (w307:string)
            n151 = Bundle By Name(cluster=T16 {"String"="", "Query func_error"={"status"=FALSE, "code"=0, "source"=""}} ("Query func (Reply Payload)"), "String"=w307) -> (w318:T16)
            n152 = case shown="True" w319 {
              tunnel: w320 -> [_ w327]
              tunnel: w318 -> [_ w326]
              frame False {
              }
              frame True {
                n153 = Send Notification(notification=w326, notifier=w327) -> ()  [unwired: 1 in, 2 out]
              }
            }
          }
          frame "query range" {
            w332 = u8 1 items=["1st Display", "2nd Display"] ("Query form Display")
            w333 = u8 0 items=["1st Display", "2nd Display"] ("Query form Display")
            n154 = Variant To Data(error in=w346, type=T12 {"Wait Notifier"=refnum, "wait for reply"=FALSE} ("query range Argument"), Variant=w344) -> (data=w342:T12, error out=w345:errorcluster)
            n155 = Unbundle By Name(w336) -> ("DMM  name"=w335:refnum<visa-resource-name>)
            n156 = call <instrlib>:"Query the Current Range.vi"("Query form Display"=w333, "VISA resource name"=w335) -> ("Return the String"=w330:string, "VISA resource name out"=w334:refnum<visa-resource-name>)  [unwired: 7 in, 1 out]
            n157 = call <instrlib>:"Query the Current Range.vi"("Query form Display"=w332, "VISA resource name"=w334) -> ("error out"=w328:errorcluster, "Return the String"=w329:string)  [unwired: 7 in, 1 out]
            n158 = Concatenate Strings(w330, w329) -> (w331:string)
            n159 = Unbundle By Name(w342) -> ("Wait Notifier"=w341:refnum<notifier>, "wait for reply"=w340:bool)
            n160 = Merge Errors(w345, w328) -> (w337:errorcluster)
            n161 = Bundle By Name(cluster=T17 {"String"="", "query range_error"={"status"=FALSE, "code"=0, "source"=""}} ("query range (Reply Payload)"), "String"=w331) -> (w339:T17)
            n162 = case shown="True" w340 {
              tunnel: w341 -> [_ w348]
              tunnel: w339 -> [_ w347]
              frame False {
              }
              frame True {
                n163 = Send Notification(notification=w347, notifier=w348) -> ()  [unwired: 1 in, 2 out]
              }
            }
          }
          frame "---Copy This Frame---" {
            # "Duplicate this frame when creating new messages.  Change this comment in the duplicated frame to describe this message."
          }
          frame "---Exit and Error Handling---" {
            # "Separator - The following cases handle errors and exit messages."
          }
          frame "Simulate MHL Error" {
            # "#DQMH_HowTo The 'Simulate MHL Error' button  illustrates how the MHL handles errors. This event is instructional in nature and can be removed."
            # "Simulate an error occurring at the MHL"
            n164 = call "Module Name--constant.vi"() -> ("Module Name"=w353:string)  [unwired: 11 in]
            n165 = xnode "Error Ring"("parameter 0"=w353) -> ("error out"=w355:errorcluster)
            n166 = Merge Errors(w357, w355) -> (w356:errorcluster)
          }
          frame "Error" {
            # "Error - Check the error message data and respond accordingly. This message is sent by the \"Error Handler\" VIs at the end of each loop in this application."
            n167 = property class="Module Admin"(reference=w367) -> ("Accessors:External Launch"=w366:bool)  [unwired: 1 in, 2 out]
            n168 = Variant To Data(error in=w374, type=errorcluster {"status"=FALSE, "code"=0, "source"=""} ("error constant"), Variant=w369) -> (data=w375:errorcluster, error out=w372:errorcluster)
            n169 = call "Error Reported.vi"("Error"=w375) -> ()  [unwired: 10 in, 1 out]
            n170 = case shown="True" w366 {
              tunnel: [w380 _] -> w365
              tunnel: w368 -> [w378 _]
              tunnel: w375 -> [w379 _]
              frame False {
                # "If the module is running standalone, then pop up an error dialog and call the \"Exit\" message."
                n171 = call <vilib>:"Simple Error Handler.vi"("error in (no error)"=w379) -> ()  [unwired: 4 in, 5 out]
                n172 = call-poly <vilib>:"Delacor_lib_QMH_Enqueue Message (poly).vi"("Priority Message? (F)"=TRUE, "Message"="Exit", "Message Queue in"=w378) -> ("error out"=w380:errorcluster)  [unwired: 7 in, 1 out]
              }
              frame True {
                # "If the module was launched externally, calling the Error Reported broadcast VI is the only action performed by the \"Error\" message. The module's caller can then process the error appropriately."
              }
            }
            n173 = Merge Errors(w372, w365) -> (w371:errorcluster)
            n174 = local write "error out"(w371) -> ()
          }
          frame "Exit" {
            w387 = 91  # 91: not all Exit messages will have an argument
            w389 = TRUE  # Stop the VI
            # "Exit - Exit the application."
            n175 = Variant To Data(error in=w396, type=T10 {"Origin"="", "Exit via Stop Module Req?"=FALSE, "Wait for Module to stop?"=FALSE} ("Stop Argument"), Variant=w388) -> (data=w385:T10, error out=w392:errorcluster)
            n176 = control-ref of="This VI"() -> (w384:refnum<vi>)
            n177 = call "Handle Exit.vi"("Stop Argument"=w385, "Admin in"=w383, "VI reference"=w384) -> ("error out"=w391:errorcluster)  [unwired: 7 in, 1 out]
            n178 = call <vilib>:"Clear Errors.vi"("error in (no error)"=w392, "specific error code to clear (0: all)"=w387) -> ("error out"=w395:errorcluster)  [unwired: 4 in, 1 out]
            n179 = disable-structure shown="NO_HARDWARE==TRUE" {
              disable-tunnel: w382 -> [w401 _]
              disable-tunnel: [w400 _] -> w381
              frame condition #0 (active) {
                n180 = Unbundle By Name(w401) -> ("DMM  name"=w399:refnum<visa-resource-name>)
                n181 = call <instrlib>:"Reset.vi"("VISA resource name"=w399) -> ("error out"=w397:errorcluster, "VISA resource name out"=w398:refnum<visa-resource-name>)  [unwired: 9 in]
                n182 = call <instrlib>:"Close.vi"("error in (no error)"=w397, "VISA resource name"=w398) -> ("error out"=w400:errorcluster)  [unwired: 9 in]
              }
              frame condition #1 {
              }
            }
            n183 = call-dynamic "Delacor_lib_QMH_Release Message Queue.vi"("error in"=w395, "Message Queue"=w390) -> ("error out"=w394:errorcluster)  [unwired: 9 in]
            n184 = Merge Errors(w394, w391, w381) -> (w393:errorcluster)
          }
          frame Default {
            # "'Default' case only runs if there is a message that isn't defined in any of the other cases.  Output a programming error."
            n185 = call "Module Name--constant.vi"() -> ("Module Name"=w402:string)  [unwired: 11 in]
            n186 = xnode "Error Ring"("parameter 0"=w403, "parameter 1"=w402) -> ("error out"=w407:errorcluster)
            n187 = Merge Errors(w405, w407) -> (w406:errorcluster)
          }
        }
        n188 = call-dynamic "Delacor_lib_QMH_Error Handler - Message Handling Loop.vi"("error in"=w176, "Message Queue in"=w166) -> ("dup error in"=w173:errorcluster)  [unwired: 8 in, 1 out]
      }
    }
    frame Error {
      # "Synchronize Caller Events.vi will inform Start Module.vi that the module has launched and will let the code calling Start Module.vi register for broadcasts and would permit the caller receive the broadcast that an error occurred at launch time."
      n189 = call "Synchronize Caller Events.vi"("Singleton Module Admin in"=w419) -> ("error out"=w424:errorcluster)  [unwired: 9 in, 1 out]
      n190 = call-dynamic "Delacor_lib_QMH_Release Message Queue.vi"("error in"=w418, "Message Queue"=w416) -> ("error out"=w417:errorcluster)  [unwired: 9 in]
      n191 = call "Module Name--constant.vi"() -> ("Module Name"=w422:string)  [unwired: 11 in]
      n192 = Merge Errors(w417, w424) -> (w425:errorcluster)
      n193 = Format Into String(format string="An error occurred during initialization. %s is no longer running.", w422) -> (resulting string=w420:string)  [unwired: 2 in, 1 out]
      n194 = call "Error Reported.vi"("Additional Information"=w420, "Error"=w425) -> ()  [unwired: 9 in, 1 out]
    }
  }
  n195 = Merge Errors(w14, w17) -> (w13:errorcluster)
  n196 = call "Close Module.vi"("error in (no error)"=w13, "Module Admin in"=w8) -> ("error out"=w15:errorcluster, "External Launch"=w1:bool, "Module Admin out"=w2:refnum<class "Delacor_lib_QMH_Module Admin.lvclass">)  [unwired: 7 in]
  n197 = Unregister For Events(event registration refnum=w7, error in=w15) -> (error out=w12:errorcluster)
  "error out" <- w12
  n198 = local write "Module Admin"(w2) -> ()
  n199 = case "External Launch?" shown="False" w1 {
    tunnel: w12 -> [_ w426]
    frame False {
    }
    frame True {
      n200 = case shown="Error" w426 {
        frame No Error {
          n201 = invoke class="VI" method="FP.Close"() -> ()  [unwired: 3 in, 3 out]
        }
        frame Error {
          n202 = invoke class="VI" method="FP.Open"("Activate"=TRUE ("Activate?")) -> ()  [unwired: 4 in, 5 out]
        }
      }
    }
  }
